vi "launch_service.vi"(8 "error in (no error)":errorcluster, 11 "system.logging in":refnum<class "system.logging.lvclass">) -> (0 "error out":errorcluster, 3 "system.logging out":refnum<class "system.logging.lvclass">)   [LabVIEW 2021, in "system.logging.lvclass"]
uses:
  system.logging.lvclass
  system.logging.lvclass/system.logging.ctl
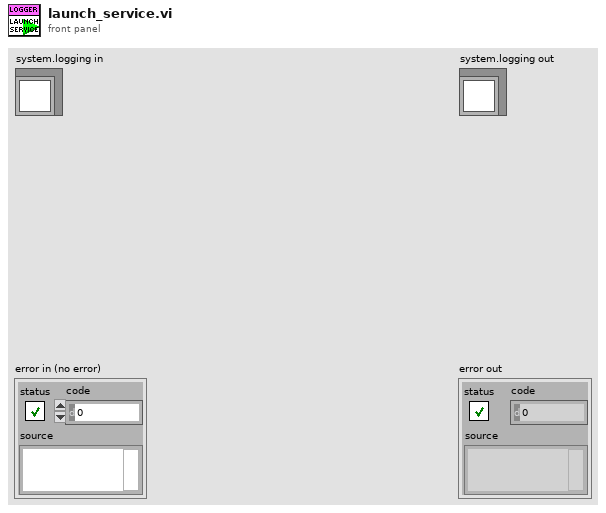
[diagram p1: front panel]
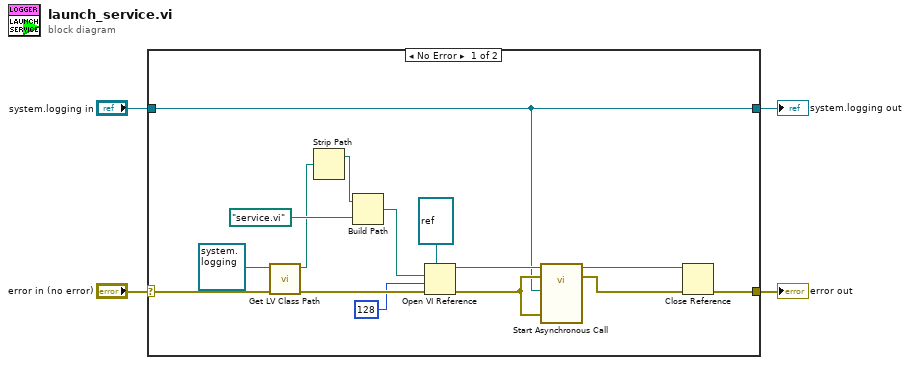
[diagram p0: block diagram]
diagram:
  n1 = case shown="No Error" "error in (no error)" {
    selector: "error in (no error)" -> [w19 w21]
    tunnel: [w5 w21] -> w3
    tunnel: [w8 w20] -> w1
    tunnel: "system.logging in" -> [w8 w20]
    frame No Error {
      n2 = call <vilib>:"Get LV Class Path.vi"("error in (no error)"=w19, "object"=refnum<class "system.logging.lvclass"> refnum ("system.logging.lvclass")) -> ("error out"=w17:errorcluster, "class path"=w12:path)  [unwired: 8 in]
      n3 = Strip Path(path=w12) -> (stripped path=w11:path)  [unwired: 1 out]
      n4 = Build Path(base path=w11, name or relative path=path "service.vi") -> (appended path=w15:path)
      n5 = Open VI Reference(type specifier VI Refnum (for type only)=refnum<vi> refnum, vi path=w15, options=128, error in (no error)=w17) -> (vi reference=w9:refnum<vi>, error out=w14:errorcluster)  [unwired: 2 in]
      n6 = call-by-ref "Start Asynchronous Call"(reference=w9, error in=w14, 8:"error in (no error)"=w14, "system.logging in"=w8) -> (reference out=w7:refnum<vi>, error out=w6:errorcluster)  [unwired: 9 in, 1 out]
      n7 = Close Reference(reference=w7, error in (no error)=w6) -> (error out=w5:errorcluster)
    }
    frame Error {
    }
  }
  "error out" <- w3
  "system.logging out" <- w1
